vi "RGB2Temperature.vi"(1 "低温？":bool, 2 "B":u8, 3 "G":u8, 4 "R":u8) -> (0 "Temperature":dbl)   [LabVIEW 2012]
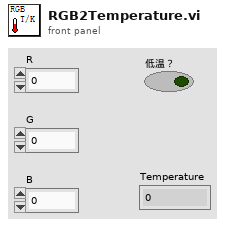
[diagram p1: front panel]
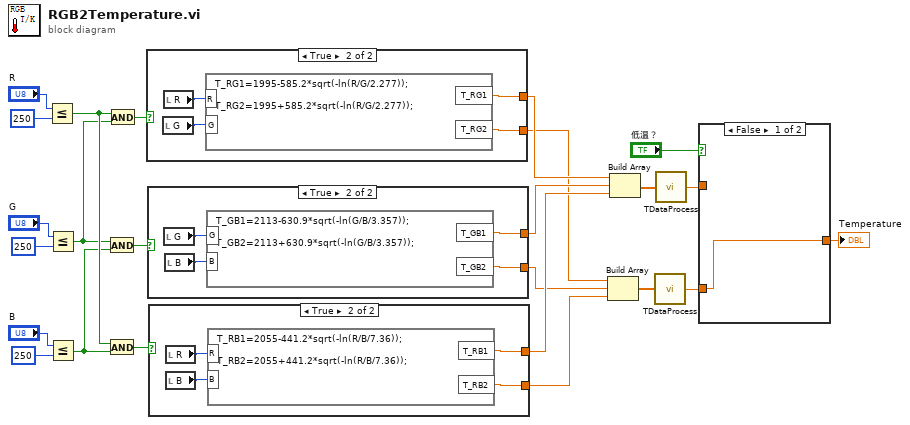
[diagram p0: block diagram]
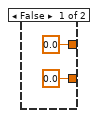
[diagram p2: hidden frame]
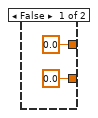
[diagram p3: hidden frame]
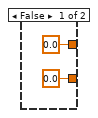
[diagram p4: hidden frame]
diagram:
  n1 = Less Or Equal?(x="R", y=u8 250) -> (x <= y?=w11:bool)
  n2 = Less Or Equal?(x="G", y=u8 250) -> (x <= y?=w10:bool)
  n3 = Less Or Equal?(x="B", y=u8 250) -> (x <= y?=w9:bool)
  n4 = And(x=w10, y=w9) -> (x .and. y?=w8:bool)
  n5 = And(x=w11, y=w9) -> (x .and. y?=w7:bool)
  n6 = And(x=w11, y=w10) -> (x .and. y?=w12:bool)
  n7 = case shown="True" w12 {
    tunnel: [0.0 ("T_RG1") w28] -> w6
    tunnel: [0.0 ("T_RG2") w27] -> w3
    frame False {
    }
    frame True {
      n8 = local read "G"() -> (w30:u8)
      n9 = local read "R"() -> (w29:u8)
      n10 = formula code="T_RG1=1995-585.2*sqrt(-ln(R/G/2.277));\n\nT_RG2=1995+585.2*sqrt(-ln(R/G/2.277));"("G"=w30, "R"=w29) -> ("T_RG1"=w28:dbl, "T_RG2"=w27:dbl)
    }
  }
  n11 = case shown="True" w8 {
    tunnel: [0.0 ("T_GB1") w34] -> w5
    tunnel: [0.0 ("T_GB2") w33] -> w2
    frame False {
    }
    frame True {
      n12 = local read "G"() -> (w35:u8)
      n13 = local read "B"() -> (w36:u8)
      n14 = formula code="T_GB1=2113-630.9*sqrt(-ln(G/B/3.357));\n\nT_GB2=2113+630.9*sqrt(-ln(G/B/3.357));"("B"=w36, "G"=w35) -> ("T_GB1"=w34:dbl, "T_GB2"=w33:dbl)
    }
  }
  n15 = case shown="True" w7 {
    tunnel: [0.0 ("T_RB1") w40] -> w4
    tunnel: [0.0 ("T_RB2") w39] -> w1
    frame False {
    }
    frame True {
      n16 = local read "R"() -> (w41:u8)
      n17 = local read "B"() -> (w42:u8)
      n18 = formula code="T_RB1=2055-441.2*sqrt(-ln(R/B/7.36));\n\nT_RB2=2055+441.2*sqrt(-ln(R/B/7.36));"("B"=w42, "R"=w41) -> ("T_RB1"=w40:dbl, "T_RB2"=w39:dbl)
    }
  }
  n19 = Build Array(w3, w2, w1) -> (w20:dbl[])
  n20 = Build Array(w6, w5, w4) -> (w22:dbl[])
  n21 = call "TDataProcess.vi"("温度数组"=w20) -> ("温度值"=w19:dbl)
  n22 = call "TDataProcess.vi"("温度数组"=w22) -> ("温度值"=w21:dbl)
  n23 = case shown="False" "低温？" {
    tunnel: w21 -> [_ w44]
    tunnel: w19 -> [w43 _]
    tunnel: [w43 w44] -> w23
    frame False {
    }
    frame True {
    }
  }
  "Temperature" <- w23
